vi "数据显示界面(子VI).vi"(0 "数据数组":string[][](array[string])) -> ()   [LabVIEW 2016]
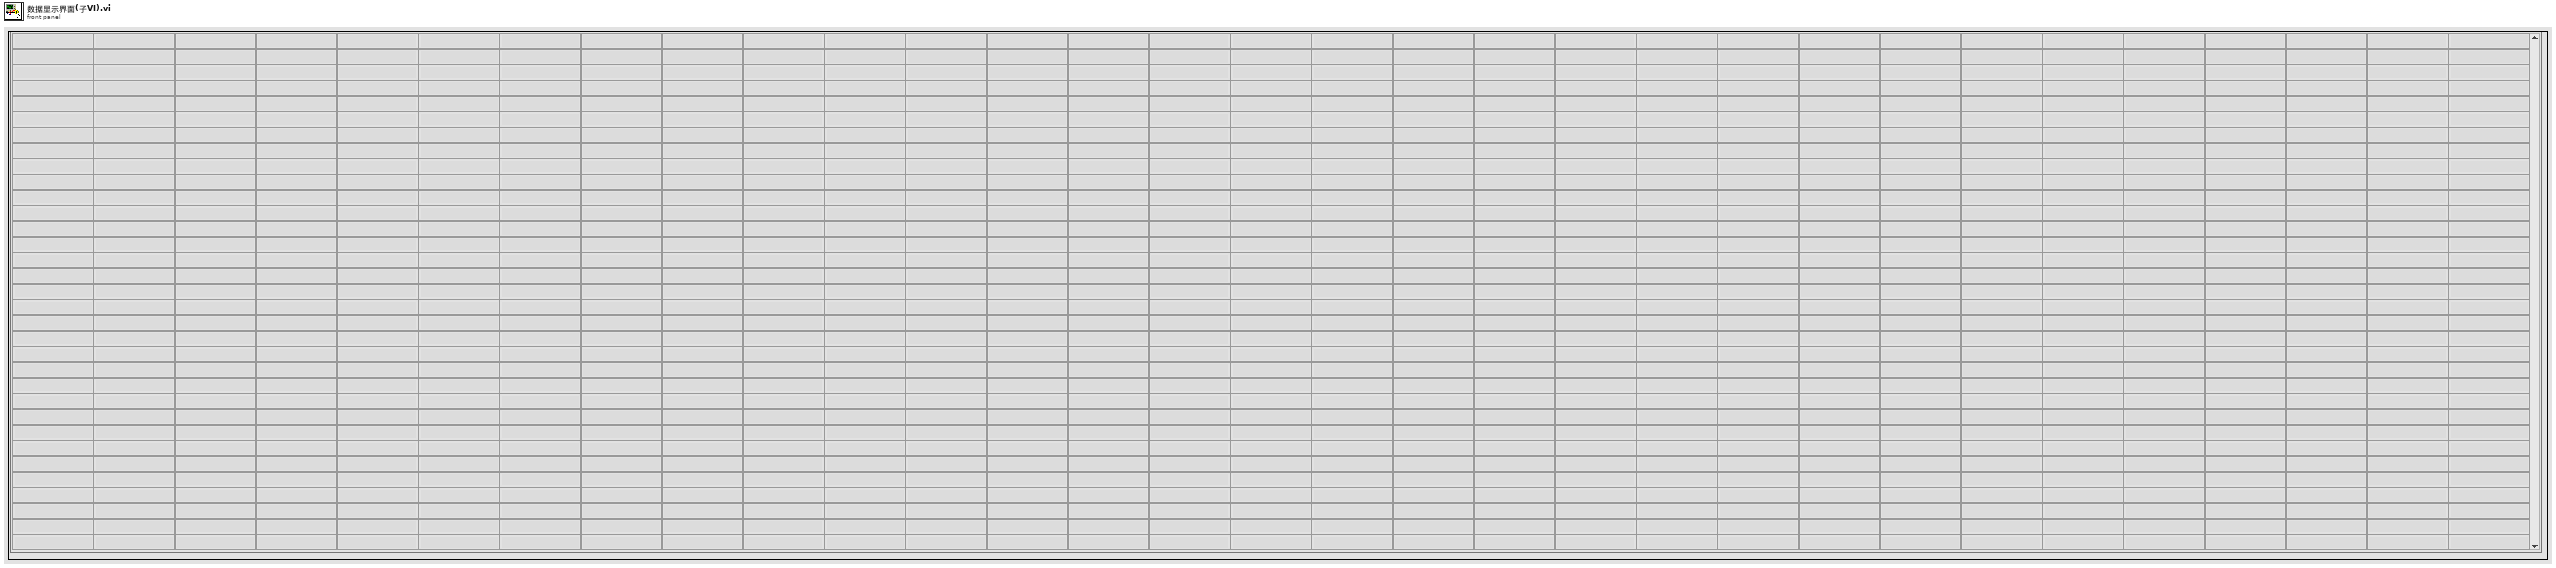
[diagram p1: front panel]
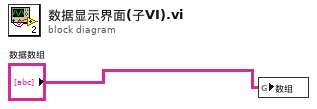
[diagram p0: block diagram]
diagram:
  n1 = global write "数据显示.vi" "数组"("数据数组") -> ()
